vi "Logger_Loop.vi"(8 "error in (no error)":errorcluster, 11 "Logger Loop Cluster in":T1) -> (0 "error out":errorcluster, 3 "Logger Cluster out":T1)   [LabVIEW 2016]
uses:
  Logger Cluster.ctl
  Classes/DataLogger/Data Logger.lvclass
  Classes/CAlex2/TypeDef/CAlexVersion.ctl
  <vilib>/Platform/TimedLoop/XDataNode/timing_clust.ctl
  <vilib>/Platform/TimedLoop/XDataNode/nitl_modes.ctl
  <vilib>/Platform/TimedLoop/XDataNode/wakeup.ctl
  <vilib>/DAQmx/read.llb/DAQmx Read (Digital Bool 1Line 1Point).vi
  <vilib>/DAQmx/write.llb/DAQmx Write (Digital Bool 1Line 1Point).vi
  GlobalVariables/Path_GV.vi
  <vilib>/DAQmx/miscellaneous.llb/DAQmx Fill In Error Info.vi
  <vilib>/Platform/TimedLoop/XDataNode/XDataNode.xnode
  <vilib>/Platform/TimedLoop/XDataNode/XDNodeRunTimeDep.lvlib
  <vilib>/AuZn/auzn custom VIs/AuZnCustomVI.lvlib
  Classes/CAlex2/CAlex2.lvclass
panel:
  out "SyncOut":bool=TRUE
  in  "PulseSyncOut":bool
  out "Starting Column of Each Variable":i32[](array[numeric])
  out "Number of Columns":i32
  out "StartTime":dbl
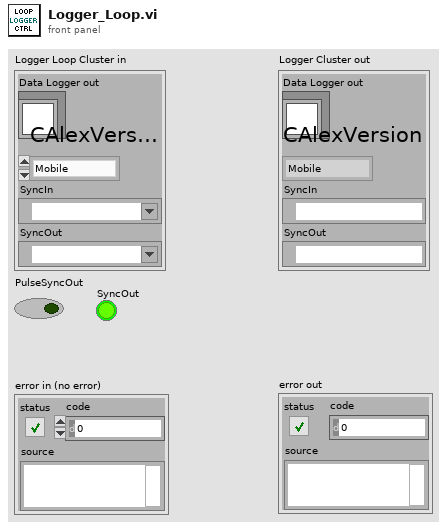
[diagram p1: front panel]
types:
  T1 = typedef "Logger Cluster.ctl" = cluster{"Data Logger out":refnum<class "Data Logger.lvclass">, "CAlexVersion":T2, "SyncIn":refnum<k21>, "SyncOut":refnum<k21>}
  T2 = typedef "CAlex2.lvclass/CAlexVersion.ctl" = enum16{"Mobile", "MobileLeft\n", "Treadmill", "Treadmill Left\n"}
  T3 = enum16{"Idle", "CloseFile", "WriteFile", "CreateFile"}
  T4 = typedef "XDNodeRunTimeDep.lvlib/timing_clust.ctl" = cluster{"Expected End [f-1]":u64, "Actual End [f-1]":u64, "Finished Late? [f-1]":bool, "Expected End [i-1]":u64, "Actual End [i-1]":u64, "Finished Late? [i-1]":bool, "Expected Start [i]":u64, "Actual Start [i]":u64, "Expected Start [f]":u64, "Actual Start [f]":u64, "Source Name":string, "Structure Name":string, "Period":i64, "Deadline":i64, "Offset":i64, "Start":i64, "Priority":i32, "Timeout":i32, "Mode":T5, "Wakeup Reason":T6, "Error":errorcluster, "Source Type":string, "Secondary Source Type":string, "Global End Time":u64, "Global Start Time":u64, "Frame Duration":u64, "Iteration Duration":u64, "Assigned CPU":i32, "I/O Scan Engine Mode":u32}
  T5 = typedef "XDNodeRunTimeDep.lvlib/nitl_modes.ctl" = enum32{"No Change", "Process missed periods, maintain original phase", "Discard missed periods, maintain original phase", "Process missed periods, ignore original phase", "Discard missed periods, ignore original phase"}
  T6 = typedef "XDNodeRunTimeDep.lvlib/wakeup.ctl" = enum32{"Normal", "Aborted", "Asynchronous wakeup", "Timing source error", "Timed loop error", "Timeout"}
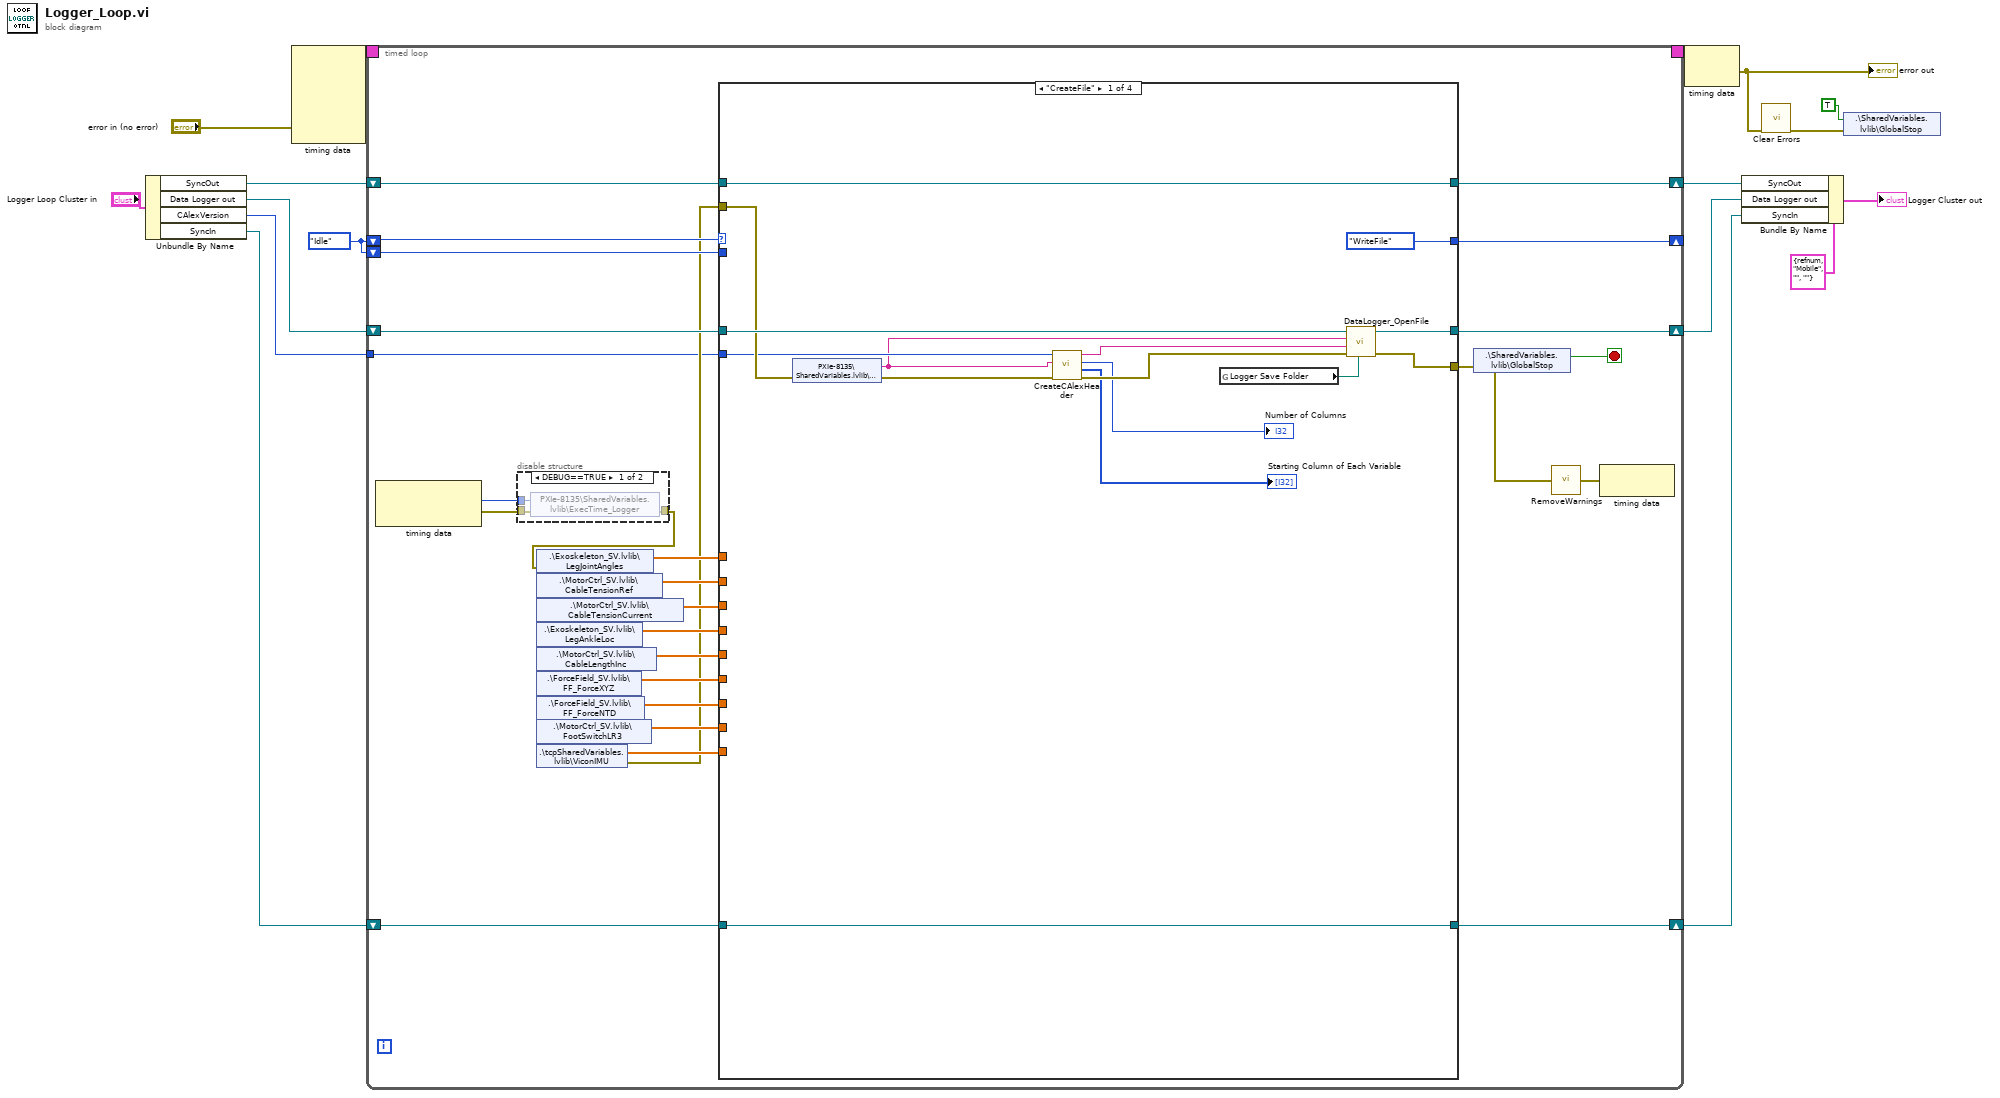
[diagram p0: block diagram]
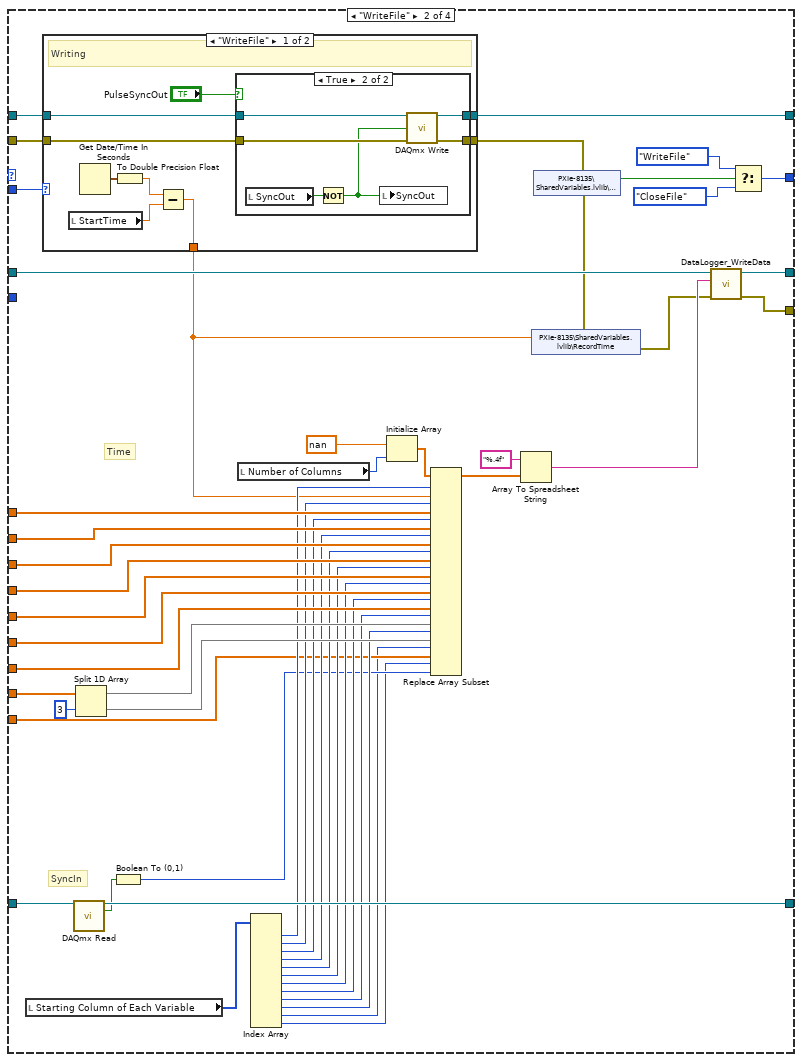
[diagram p3: hidden frame]
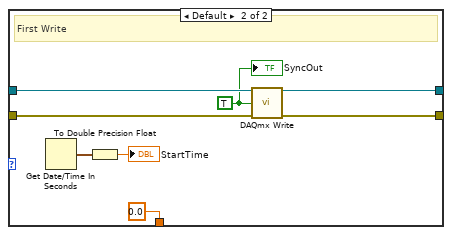
[diagram p5: hidden frame]
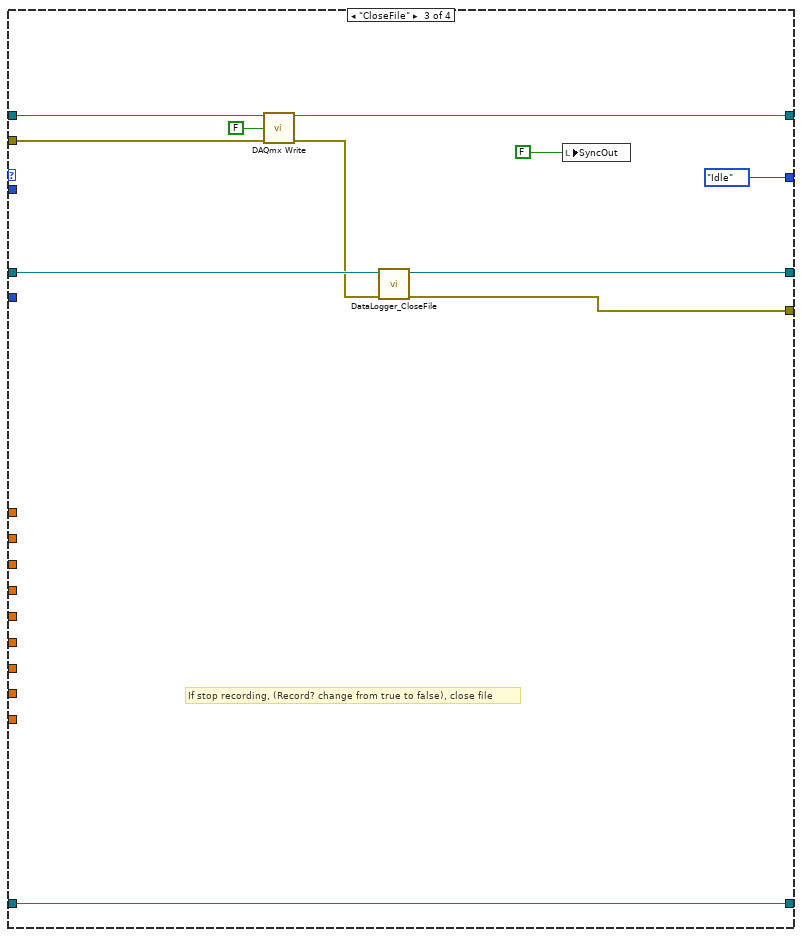
[diagram p6: hidden frame]
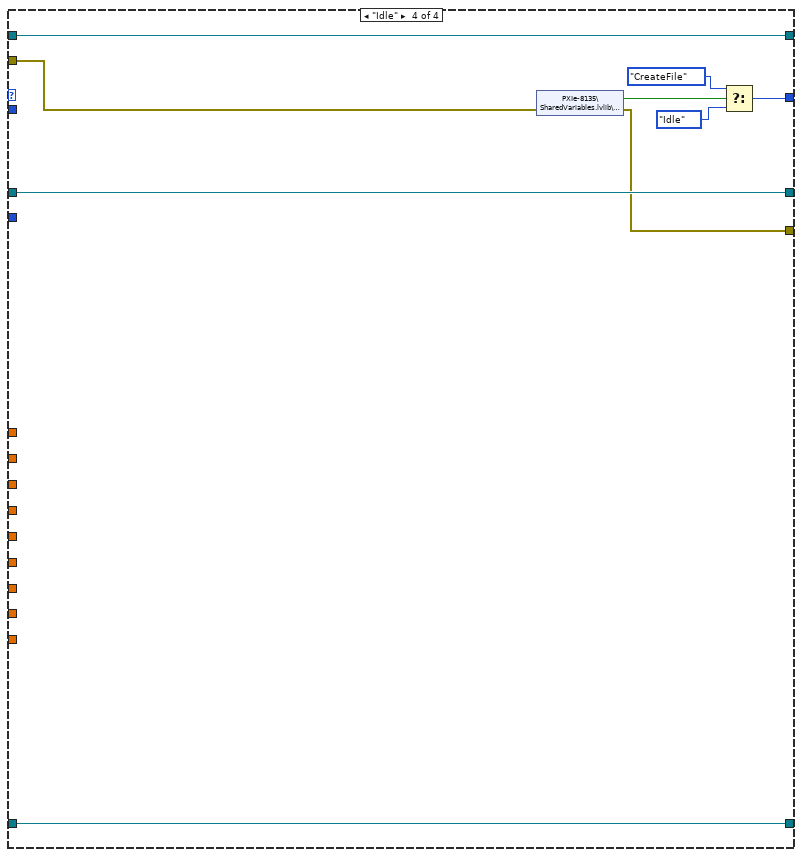
[diagram p7: hidden frame]
diagram:
  w15 = T3."Idle"
  n1 = Unbundle By Name("Logger Loop Cluster in") -> ("SyncOut"=w9:refnum<k21>, "Data Logger out"=w2:refnum<class "Data Logger.lvclass">, "CAlexVersion"=w1:T2, "SyncIn"=w8:refnum<k21>)
  n2 = node-c288("error in (no error)") -> (w17:T4)  [unwired: 4 in]
  n3 = timed-loop {
    timing: w17 -> [_]
    timing-out: [_] -> w16
    shift-right: [w51] -> w3
    shift-left: w2 -> [w52]
    shift-right: [w44] -> _
    shift-left: w15 -> [w43]
    shift-left: w15 -> [w29]
    shift-right: [w34] -> w4
    shift-left: w9 -> [w35]
    shift-right: [w30] -> w6
    shift-left: w8 -> [w31]
    tunnel: w1 -> [w18]
    stop <- w27 stop-if-true
    n4 = node-c288() -> (w28:i64, w25:errorcluster)  [unwired: 1 in]
    n5 = disable-structure shown="DEBUG==TRUE" {
      disable-tunnel: w28 -> [w55 _]
      disable-tunnel: w25 -> [w54 w56]
      disable-tunnel: [w53 w56] -> w24
      frame condition #0 {
        n6 = shared-variable "PXIe-8135\\SharedVariables.lvlib\\ExecTime_Logger"(w55, error in=w54) -> (error out=w53:errorcluster)
      }
      frame condition #1 (active) {
      }
    }
    n7 = shared-variable ".\\Exoskeleton_SV.lvlib\\LegJointAngles"(error in=w24) -> (w45:dbl[], error out=w41:errorcluster)
    n8 = shared-variable ".\\MotorCtrl_SV.lvlib\\CableTensionRef"(error in=w41) -> (w46:dbl[], error out=w40:errorcluster)
    n9 = shared-variable ".\\MotorCtrl_SV.lvlib\\CableTensionCurrent"(error in=w40) -> (w47:dbl[], error out=w39:errorcluster)
    n10 = shared-variable ".\\Exoskeleton_SV.lvlib\\LegAnkleLoc"(error in=w39) -> (w48:dbl[], error out=w38:errorcluster)
    n11 = shared-variable ".\\MotorCtrl_SV.lvlib\\CableLengthInc"(error in=w38) -> (w42:dbl[], error out=w36:errorcluster)
    n12 = shared-variable ".\\ForceField_SV.lvlib\\FF_ForceXYZ"(error in=w36) -> (w49:dbl[], error out=w37:errorcluster)
    n13 = shared-variable ".\\ForceField_SV.lvlib\\FF_ForceNTD"(error in=w37) -> (w50:dbl[], error out=w33:errorcluster)
    n14 = shared-variable ".\\MotorCtrl_SV.lvlib\\FootSwitchLR3"(error in=w33) -> (w32:dbl[], error out=w21:errorcluster)
    n15 = shared-variable ".\\tcpSharedVariables.lvlib\\ViconIMU"(error in=w21) -> (w20:dbl[], error out=w19:errorcluster)
    n16 = case shown="\"CreateFile\"" w43 {
      tunnel: w52 -> [w71 w112 w157 w166]
      tunnel: w19 -> [w70 w105 w153 w159]
      tunnel: [w68 w121 w149 w166] -> w51
      tunnel: [w60 w120 w148 w158] -> w26
      tunnel: w50 -> [_ w107 _ _]
      tunnel: w49 -> [_ w108 _ _]
      tunnel: w42 -> [_ w117 _ _]
      tunnel: w48 -> [_ w116 _ _]
      tunnel: w47 -> [_ w115 _ _]
      tunnel: w46 -> [_ w114 _ _]
      tunnel: w45 -> [_ w113 _ _]
      tunnel: [T3."WriteFile" w109 T3."Idle" w163] -> w44
      tunnel: w35 -> [w64 w106 w155 w162]
      tunnel: [w64 w104 w154 w162] -> w34
      tunnel: w32 -> [_ w95 _ _]
      tunnel: w31 -> [w63 w103 w150 w161]
      tunnel: [w63 w102 w150 w161] -> w30
      tunnel: w29 -> [_ w81 _ _]
      tunnel: w20 -> [_ w78 _ _]
      tunnel: w18 -> [w58 _ _ _]
      frame "CreateFile" {
        n17 = shared-variable "PXIe-8135\\SharedVariables.lvlib\\FileName"(error in=w70) -> (w57:string, error out=w66:errorcluster)
        n18 = call "CreateCAlexHeader.vi"("error in (no error)"=w66, "FileName"=w57, "CAlexVersion"=w58) -> ("error out"=w65:errorcluster, "Starting Columns of Each Variable"=→"Starting Column of Each Variable":i32[], "Number of Columns"=→"Number of Columns":i32, "header"=w69:string)  [unwired: 5 in]
        n19 = global read "Path_GV.vi" "Logger Save Folder"() -> (w59:path)
        n20 = call "DataLogger_OpenFile.vi"("base path (C:\\CAlex\\)"=w59, "error in (no error)"=w65, "Header"=w69, "File Name"=w57, "Data Logger in"=w71) -> ("error out"=w60:errorcluster, "Data Logger out"=w68:refnum<class "Data Logger.lvclass">)  [unwired: 5 in]
      }
      frame "WriteFile" {
        # "Time"
        # "SyncIn"
        n21 = local read "Starting Column of Each Variable"() -> (w96:i32[])
        n22 = case shown="\"WriteFile\"" w81 {
          tunnel: w106 -> [w125 w146]
          tunnel: w105 -> [w123 w145]
          tunnel: [w122 w144] -> w73
          tunnel: [w124 w143] -> w104
          tunnel: [w127 0.0 ("StartTime")] -> w80
          frame "WriteFile" {
            # "Writing"
            n23 = local read "StartTime"() -> (w128:dbl)
            n24 = Get Date/Time In Seconds() -> (seconds since 1Jan1904=w130:timestamp)
            n25 = To Double Precision Float(number=w130) -> (double precision float=w129:dbl)
            n26 = Subtract(x=w129, y=w128) -> (x-y=w127:dbl)
            n27 = case shown="True" "PulseSyncOut" {
              tunnel: w125 -> [w132 w138]
              tunnel: [w132 w137] -> w124
              tunnel: w123 -> [w131 w136]
              tunnel: [w131 w135] -> w122
              frame False {
              }
              frame True {
                n28 = local read "SyncOut"() -> (w134:bool)
                n29 = Not(x=w134) -> (.not. x?=w133:bool)
                n30 = local write "SyncOut"(w133) -> ()
                n31 = call-poly <vilib>:"DAQmx Write.vi"("task/channels in"=w138, "data"=w133, "error in"=w136) -> ("task out"=w137:refnum<k21>, "error out"=w135:errorcluster)  [unwired: 10 in, 1 out]
              }
            }
          }
          frame Default {
            w142 = TRUE ("data")
            # "First Write"
            n32 = Get Date/Time In Seconds() -> (seconds since 1Jan1904=w141:timestamp)
            n33 = To Double Precision Float(number=w141) -> (double precision float=→"StartTime":dbl)
            n34 = call-poly <vilib>:"DAQmx Write.vi"("task/channels in"=w146, "data"=w142, "error in"=w145) -> ("task out"=w143:refnum<k21>, "error out"=w144:errorcluster)  [unwired: 10 in, 1 out]
            "SyncOut" <- w142
          }
        }
        n35 = call-poly <vilib>:"DAQmx Read.vi"("task/channels in"=w103) -> ("task out"=w102:refnum<k21>, "data"=w101:bool)  [unwired: 12 in, 1 out]
        n36 = Split 1D Array(array=w95, index=3) -> (first subarray=w94:dbl[], second subarray=w93:dbl[])
        n37 = Boolean To (0,1)(Boolean=w101) -> (0, 1=w77:i16)
        n38 = local read "Number of Columns"() -> (w97:i32)
        n39 = Index Array(array=w96) -> (element #1=w91:i32, element #2=w90:i32, element #3=w89:i32, element #4=w88:i32, element #5=w87:i32, element #6=w86:i32, element #7=w85:i32, element #8=w84:i32, element #9=w83:i32, element #10=w82:i32, element #11=w76:i32, element #12=w75:i32)  [unwired: 12 in]
        n40 = Initialize Array(nan ("element"), w97) -> (w119:dbl[])
        n41 = Replace Array Subset(array=w119, new element #1=w80, index #1=w91, new element #2=w113, index #2=w90, new element #3=w114, index #3=w89, new element #4=w115, index #4=w88, new element #5=w116, index #5=w87, new element #6=w117, index #6=w86, new element #7=w108, index #7=w85, new element #8=w107, index #8=w84, new element #9=w94, index #9=w83, new element #10=w93, index #10=w82, new element #11=w78, index #11=w76, new element #12=w77, index #12=w75) -> (w100:dbl[])
        n42 = Array To Spreadsheet String(array=w100, 3:"%.4f" ("format string")) -> (spreadsheet string=w99:string)  [unwired: 1 in]
        n43 = shared-variable "PXIe-8135\\SharedVariables.lvlib\\Record?"(error in=w73) -> (w74:bool, error out=w72:errorcluster)
        n44 = shared-variable "PXIe-8135\\SharedVariables.lvlib\\RecordTime"(w80, error in=w72) -> (error out=w79:errorcluster)
        n45 = call "DataLogger_WriteData.vi"("error in (no error)"=w79, "New line"=w99, "Data Logger in"=w112) -> ("error out"=w120:errorcluster, "Data Logger out"=w121:refnum<class "Data Logger.lvclass">)  [unwired: 7 in]
        n46 = Select(t=T3."WriteFile", s=w74, f=T3."CloseFile") -> (s? t:f=w109:T3)
      }
      frame "CloseFile" {
        # "If stop recording, (Record? change from true to false), close file"
        n47 = call-poly <vilib>:"DAQmx Write.vi"("task/channels in"=w155, "data"=FALSE, "error in"=w153) -> ("task out"=w154:refnum<k21>, "error out"=w152:errorcluster)  [unwired: 10 in, 1 out]
        n48 = call "DataLogger_CloseFile.vi"("error in (no error)"=w152, "Data Logger in"=w157) -> ("error out"=w148:errorcluster, "Data Logger out"=w149:refnum<class "Data Logger.lvclass">)  [unwired: 8 in]
        n49 = local write "SyncOut"(FALSE ("SyncOut")) -> ()
      }
      frame "Idle" {
        n50 = shared-variable "PXIe-8135\\SharedVariables.lvlib\\Record?"(error in=w159) -> (w160:bool, error out=w158:errorcluster)
        n51 = Select(t=T3."CreateFile", s=w160, f=T3."Idle") -> (s? t:f=w163:T3)
      }
    }
    n52 = shared-variable ".\\SharedVariables.lvlib\\GlobalStop"(error in=w26) -> (w27:bool, error out=w22:errorcluster)
    n53 = call <vilib>:"RemoveWarnings.vi"("error in (no error)"=w22) -> ("error out"=w23:errorcluster)
    n54 = node-c288(w23) -> ()  [unwired: 1 out]
  }
  n55 = node-c288(w16) -> (w13:errorcluster)
  "error out" <- w13
  n56 = Bundle By Name(cluster=T1 {"Data Logger out"=refnum, "CAlexVersion"=enum."Mobile", "SyncIn"="", "SyncOut"=""} ("Logger Loop Cluster out"), "SyncOut"=w4, "Data Logger out"=w3, "SyncIn"=w6) -> (→"Logger Cluster out":T1)
  n57 = call <vilib>:"Clear Errors.vi"("error in (no error)"=w13) -> ("error out"=w12:errorcluster)  [unwired: 5 in, 1 out]
  n58 = shared-variable ".\\SharedVariables.lvlib\\GlobalStop"(TRUE ("GlobalStop"), error in=w12) -> ()  [unwired: 1 out]
